vi "process_DAQ_NI.vi"(8 "error in (no error)":errorcluster) -> (0 "error out":errorcluster)   [LabVIEW 2010]
uses:
  typedefs/control_daq_enum.ctl
  typedefs/data_cluster.ctl
  typedefs/control_shutter_enum.ctl
  typedefs/main_state_enum.ctl
  typedefs/device_parameters.ctl
  typedefs/free_run_parameters.ctl
  typedefs/protocol_parameters.ctl
  <vilib>/DAQmx/read.llb/DAQmx Read (Analog 2D DBL NChan NSamp).vi
  <vilib>/daqmx/miscellaneous.llb/DAQmx Fill In Error Info.vi
panel:
  out "Onset":bool
  out "Waiting for trigger":bool
  out "Time [s]":dbl
  out "Repetition":dbl
  out "OFF":bool
  out "Post ON":bool
  out "ON":bool
  out "Pre ON":bool
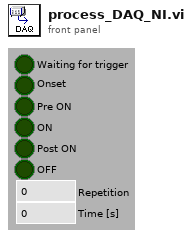
[diagram p1: front panel]
types:
  T1 = typedef "control_daq_enum.ctl" = enum16{"Init", "FreeRun", "Protocol", "Stop", "Quit"}
  T2 = cluster{"Control DAQ Enum":T1, "variant":variant}
  T3 = typedef "control_shutter_enum.ctl" = enum16{"Init", "Open", "Close", "Quit"}
  T4 = cluster{"Control shutter enum":T3, "variant":variant}
  T5 = typedef "data_cluster.ctl" = cluster{"t0":dbl, "dt":dbl, "Channels":dbl[][]}
  T6 = typedef "main_state_enum.ctl" = enum16{"Init", "Empty", "ParamsChanged", "Start", "Stop", "Abort", "Acquisition finished", "SetShutter", "Reset", "Error", "Quit"}
  T7 = typedef "device_parameters.ctl" = cluster{"Triggered?":bool, "Shutter channel":tag, "Acquisition channels":tag, "Acquisition sample rate":dbl, "Read chunk size":i32, "Stimulation channel":tag, "Stimulation sample rate":dbl}
  T8 = typedef "free_run_parameters.ctl" = cluster{"Stim onset":dbl, "Stim frequency":dbl, "Stim length":dbl, "Sync shutter to acquisition":bool}
  T9 = cluster{"Device parameters":T7, "Free run parameters":T8}
  T10 = typedef "protocol_parameters.ctl" = cluster{"Repetitions":dbl, "ON time":dbl, "OFF time":dbl, "Stim onset":dbl, "Stim frequency":dbl, "Pulse width":dbl, "Acquire before ON":dbl, "Acquire after ON":dbl, "Sync shutter to acquisition":bool}
  T11 = cluster{"Device parameters":T7, "Protocol parameters":T10}
  T12 = typedef "where_in_protocol_cluster.ctl" = cluster{"Onset":bool, "PreON":bool, "ON":bool, "PostON":bool, "OFF":bool, "Repetition":dbl, "Time":dbl}
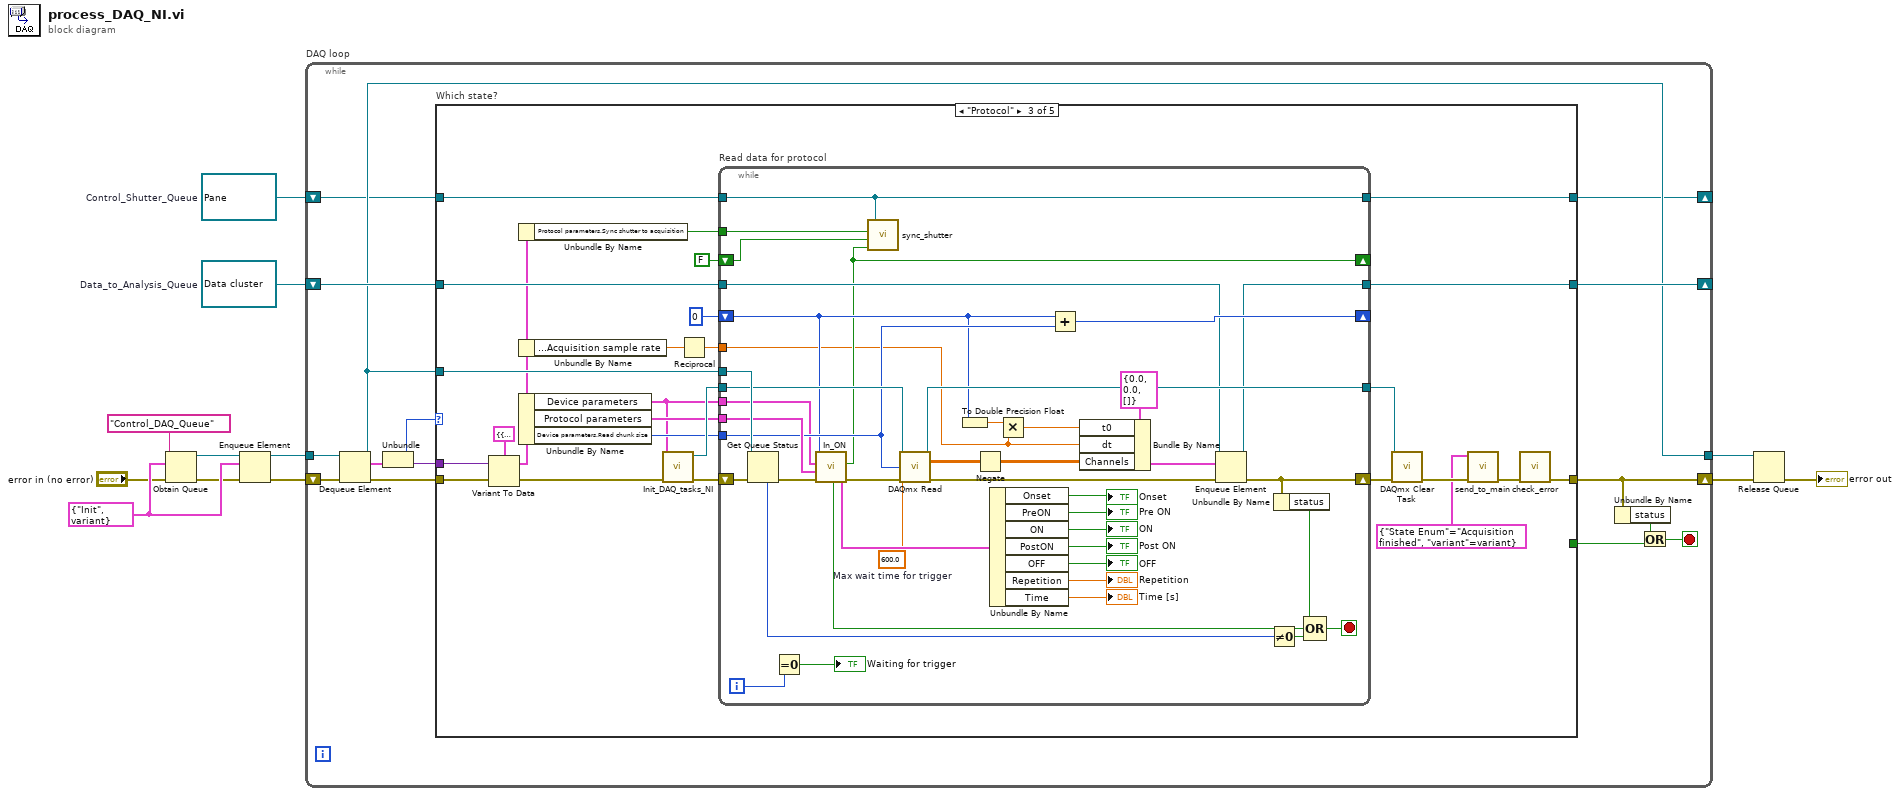
[diagram p0: block diagram]
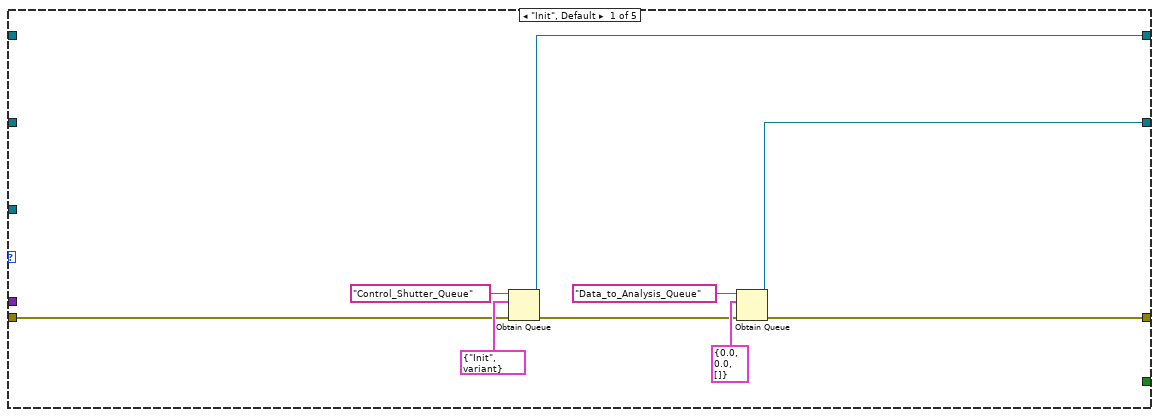
[diagram p2: hidden frame]
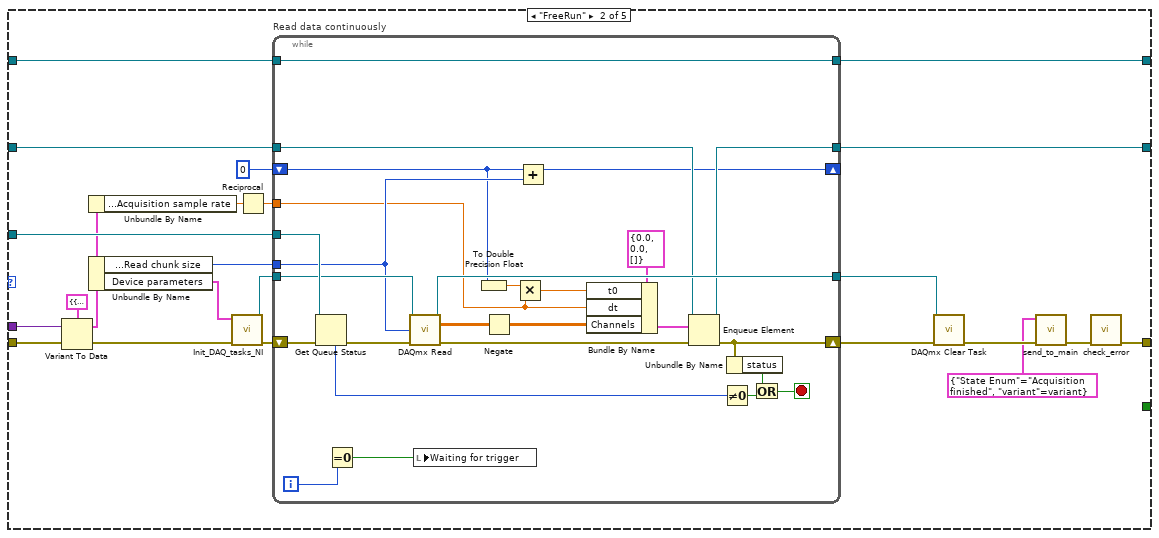
[diagram p3: hidden frame]
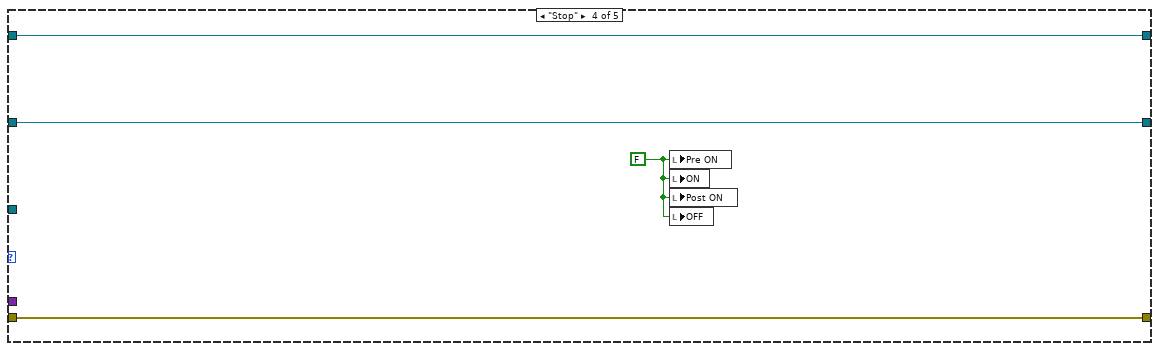
[diagram p4: hidden frame]
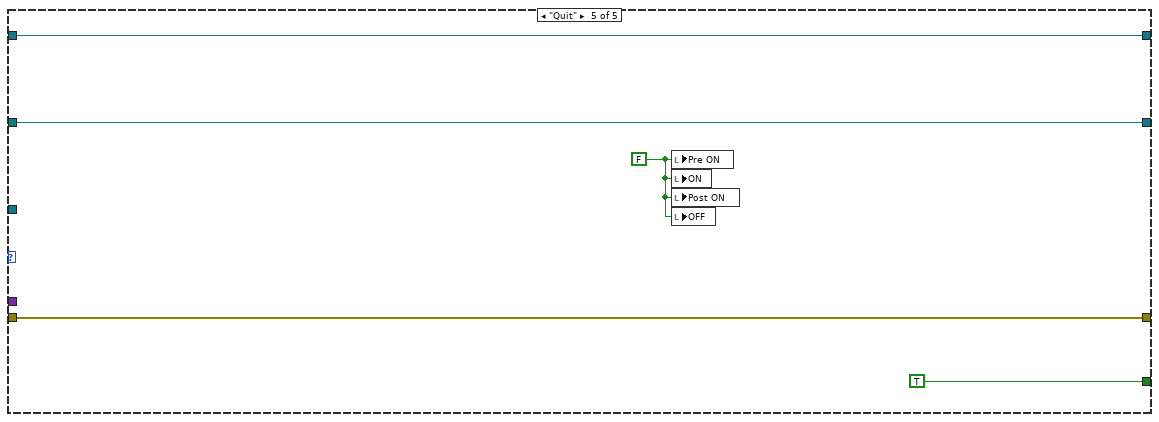
[diagram p5: hidden frame]
diagram:
  w1 = refnum<queue> refnum  # Control_Shutter_Queue
  w2 = refnum<queue> refnum  # Data_to_Analysis_Queue
  w12 = T2 {"Control DAQ Enum"=enum."Init", "variant"=variant} ("ControlDAQ state cluster")
  n1 = Obtain Queue(name (unnamed)="Control_DAQ_Queue", element data type=w12, error in (no error)="error in (no error)") -> (queue out=w8:refnum<queue>, error out=w10:errorcluster)  [unwired: 2 in, 1 out]
  n2 = Enqueue Element(queue=w8, element=w12, error in (no error)=w10) -> (queue out=w9:refnum<queue>, error out=w11:errorcluster)  [unwired: 1 in, 1 out]
  n3 = while "DAQ loop" {
    shift-right: [w21] -> w7
    shift-left: w11 -> [w26]
    tunnel: w9 -> [w27]
    tunnel: [w15] -> w6
    shift-right: [w16] -> _
    shift-left: w2 -> [w17]
    shift-right: [w13] -> _
    shift-left: w1 -> [w14]
    stop <- w19 stop-if-true
    n4 = Dequeue Element(queue=w27, error in (no error)=w26) -> (queue out=w15:refnum<queue>, element=w25:T2, error out=w23:errorcluster)  [unwired: 1 in, 1 out]
    n5 = Unbundle(w25) -> ("Control DAQ Enum"=w18:T1, "variant"=w24:variant)
    n6 = case "Which state?" shown="\"Protocol\"" w18 {
      tunnel: w15 -> [_ w59 w111 _ _]
      tunnel: w24 -> [_ w58 w110 _ _]
      tunnel: w23 -> [w28 w57 w109 w157 w161]
      tunnel: [w35 w45 w95 w157 w161] -> w21
      tunnel: [_ _ _ _ TRUE] -> w22
      tunnel: w17 -> [_ w48 w103 w156 w160]
      tunnel: [w34 w52 w102 w156 w160] -> w16
      tunnel: w14 -> [_ w43 w94 w155 w159]
      tunnel: [w29 w44 w90 w155 w159] -> w13
      frame "Init", Default {
        n7 = Obtain Queue(name (unnamed)="Control_Shutter_Queue", element data type=T4 {"Control shutter enum"=enum."Init", "variant"=variant}, error in (no error)=w28) -> (queue out=w29:refnum<queue>, error out=w32:errorcluster)  [unwired: 2 in, 1 out]
        n8 = Obtain Queue(name (unnamed)="Data_to_Analysis_Queue", element data type=T5 {"t0"=0.0, "dt"=0.0, "Channels"=[]} ("Data cluster"), error in (no error)=w32) -> (queue out=w34:refnum<queue>, error out=w35:errorcluster)  [unwired: 2 in, 1 out]
      }
      frame "FreeRun" {
        n9 = Variant To Data(error in=w57, Variant=w58, type=T9 {"Device parameters"={"Triggered?"=FALSE, "Shutter channel"="Dev1/port1/line3", "Acquisition channels"="Dev1/ai0:2", "Acquisition sample rate"=10000.0, "Read chunk size"=10, "Stimulation channel"="", "Stimulation sample rate"=100.0}, "Free run parameters"={"Stim onset"=5.0, "Stim frequency"=1.0, "Stim length"=0.001, "Sync shutter to acquisition"=TRUE}}) -> (error out=w40:errorcluster, data=w47:T9)
        n10 = Unbundle By Name(w47) -> ("Device parameters.Acquisition sample rate"=w42:dbl)
        n11 = Unbundle By Name(w47) -> ("Device parameters.Read chunk size"=w49:i32, "Device parameters"=w50:T7)
        n12 = call "Init_DAQ_tasks_NI.vi"("error in"=w40, "Device parameters"=w50) -> ("error out"=w56:errorcluster, "DAQ task out"=w55:refnum<k21>)  [unwired: 6 in]
        n13 = Reciprocal(x=w42) -> (1/x=w41:dbl)
        n14 = while "Read data continuously" {
          shift-right: [w80] -> w54
          shift-left: w56 -> [w81]
          tunnel: w59 -> [w85]
          tunnel: w55 -> [w78]
          tunnel: [w75] -> w53
          tunnel: [w74] -> w52
          tunnel: w49 -> [w69]
          tunnel: w48 -> [w73]
          tunnel: w41 -> [w66]
          shift-right: [w70] -> _
          shift-left: 0 -> [w68]
          tunnel: [w62] -> w44
          tunnel: w43 -> [w62]
          i -> [w61]
          stop <- w82 stop-if-true
          n15 = Get Queue Status(queue=w85, error in (no error)=w81) -> (error out=w76:errorcluster, # elements in queue=w84:i32)  [unwired: 1 in, 6 out]
          n16 = Equal To 0?(x=w61) -> (x = 0?=w60:bool)
          n17 = call-poly <vilib>:"DAQmx Read.vi"("task/channels in"=w78, "number of samples per channel"=w69, "error in"=w76) -> ("task out"=w75:refnum<k21>, "data"=w64:dbl[][], "error out"=w77:errorcluster)  [unwired: 10 in]
          n18 = local write "Waiting for trigger"(w60) -> ()
          n19 = To Double Precision Float(number=w68) -> (double precision float=w67:dbl)
          n20 = Negate(x=w64) -> (-x=w63:dbl[][])
          n21 = Multiply(x=w67, y=w66) -> (x*y=w65:dbl)
          n22 = Add(x=w68, y=w69) -> (x+y=w70:i32)
          n23 = Bundle By Name(cluster=T5 {"t0"=0.0, "dt"=0.0, "Channels"=[]} ("Data cluster"), "t0"=w65, "dt"=w66, "Channels"=w63) -> (w71:T5)
          n24 = Enqueue Element(queue=w73, element=w71, error in (no error)=w77) -> (queue out=w74:refnum<queue>, error out=w80:errorcluster)  [unwired: 1 in, 1 out]
          n25 = Not Equal To 0?(x=w84) -> (x != 0?=w83:bool)
          n26 = Unbundle By Name(w80) -> ("status"=w79:bool)
          n27 = Or(x=w79, y=w83) -> (x .or. y?=w82:bool)
        }
        n28 = call <vilib>:"DAQmx Clear Task.vi"("task in"=w53, "error in"=w54) -> ("error out"=w39:errorcluster)  [unwired: 13 in]
        n29 = call "send_to_main.vi"("error in (no error)"=w39, "Main state cluster"=cluster{"State Enum":T6, "variant":variant} {"State Enum"=enum."Acquisition finished", "variant"=variant} ("element")) -> ("error out"=w38:errorcluster)  [unwired: 9 in]
        n30 = call "check_error.vi"("error in"=w38) -> ("error out"=w45:errorcluster)  [unwired: 10 in]
      }
      frame "Protocol" {
        n31 = Variant To Data(error in=w109, Variant=w110, type=T11 {"Device parameters"={"Triggered?"=FALSE, "Shutter channel"="", "Acquisition channels"="", "Acquisition sample rate"=100.0, "Read chunk size"=0, "Stimulation channel"="", "Stimulation sample rate"=0.0}, "Protocol parameters"={"Repetitions"=1.0, "ON time"=40.0, "OFF time"=120.0, "Stim onset"=5.0, "Stim frequency"=1.0, "Pulse width"=1.0, "Acquire before ON"=1.0, "Acquire after ON"=0.0, "Sync shutter to acquisition"=FALSE}}) -> (error out=w91:errorcluster, data=w93:T11)
        n32 = Unbundle By Name(w93) -> ("Protocol parameters.Sync shutter to acquisition"=w92:bool)
        n33 = Unbundle By Name(w93) -> ("Device parameters.Acquisition sample rate"=w97:dbl)
        n34 = Unbundle By Name(w93) -> ("Device parameters"=w99:T7, "Protocol parameters"=w101:T10, "Device parameters.Read chunk size"=w100:i32)
        n35 = call "Init_DAQ_tasks_NI.vi"("error in"=w91, "Device parameters"=w99) -> ("error out"=w108:errorcluster, "DAQ task out"=w107:refnum<k21>)  [unwired: 6 in]
        n36 = Reciprocal(x=w97) -> (1/x=w96:dbl)
        n37 = while "Read data for protocol" {
          shift-right: [w143] -> w106
          shift-left: w108 -> [w151]
          tunnel: w111 -> [w153]
          tunnel: w107 -> [w150]
          tunnel: [w149] -> w105
          shift-right: [w148] -> _
          shift-left: 0 -> [w138]
          tunnel: w103 -> [w147]
          tunnel: [w146] -> w102
          tunnel: w99 -> [w136]
          tunnel: w101 -> [w142]
          tunnel: w100 -> [w141]
          tunnel: w96 -> [w126]
          tunnel: w94 -> [w119]
          shift-right: [w129] -> _
          shift-left: FALSE ("Do acquire") -> [w131]
          tunnel: w92 -> [w130]
          tunnel: [w119] -> w90
          i -> [w114]
          stop <- w134 stop-if-true
          w115 = 600.0  # Max wait time for trigger
          n38 = Get Queue Status(queue=w153, error in (no error)=w151) -> (error out=w145:errorcluster, # elements in queue=w152:i32)  [unwired: 1 in, 6 out]
          n39 = Equal To 0?(x=w114) -> (x = 0?=→"Waiting for trigger":bool)
          n40 = call "In_ON.vi"("error in"=w145, "Protocol parameters"=w142, "Device parameters"=w136, "Read position"=w138) -> ("error out"=w144:errorcluster, "Finished?"=w132:bool, "Do acquire"=w129:bool, "Where"=w125:T12)  [unwired: 4 in]
          n41 = call "sync_shutter.vi"("Do acquire?"=w129, "Old acquire state"=w131, "Sync shutter to acquisition"=w130, "Control_Shutter_Queue"=w119) -> ()  [unwired: 1 in]
          n42 = call-poly <vilib>:"DAQmx Read.vi"("task/channels in"=w150, "number of samples per channel"=w141, "timeout"=w115, "error in"=w144) -> ("task out"=w149:refnum<k21>, "data"=w122:dbl[][], "error out"=w140:errorcluster)  [unwired: 9 in]
          n43 = To Double Precision Float(number=w138) -> (double precision float=w128:dbl)
          n44 = Negate(x=w122) -> (-x=w121:dbl[][])
          n45 = Unbundle By Name(w125) -> ("Onset"=→"Onset":bool, "PreON"=→"Pre ON":bool, "ON"=→"ON":bool, "PostON"=→"Post ON":bool, "OFF"=→"OFF":bool, "Repetition"=→"Repetition":dbl, "Time"=→"Time [s]":dbl)
          n46 = Multiply(x=w128, y=w126) -> (x*y=w127:dbl)
          n47 = Add(x=w138, y=w141) -> (x+y=w148:i32)
          n48 = Bundle By Name(cluster=T5 {"t0"=0.0, "dt"=0.0, "Channels"=[]} ("Data cluster"), "t0"=w127, "dt"=w126, "Channels"=w121) -> (w137:T5)
          n49 = Enqueue Element(queue=w147, element=w137, error in (no error)=w140) -> (queue out=w146:refnum<queue>, error out=w143:errorcluster)  [unwired: 1 in, 1 out]
          n50 = Not Equal To 0?(x=w152) -> (x != 0?=w133:bool)
          n51 = Unbundle By Name(w143) -> ("status"=w135:bool)
          n52 = Compound Arithmetic op=OR(w135, w132, w133) -> (w134:bool)
        }
        n53 = call <vilib>:"DAQmx Clear Task.vi"("task in"=w105, "error in"=w106) -> ("error out"=w88:errorcluster)  [unwired: 13 in]
        n54 = call "send_to_main.vi"("error in (no error)"=w88, "Main state cluster"=cluster{"State Enum":T6, "variant":variant} {"State Enum"=enum."Acquisition finished", "variant"=variant} ("element")) -> ("error out"=w87:errorcluster)  [unwired: 9 in]
        n55 = call "check_error.vi"("error in"=w87) -> ("error out"=w95:errorcluster)  [unwired: 10 in]
      }
      frame "Stop" {
        w154 = FALSE ("Pre ON")
        n56 = local write "Pre ON"(w154) -> ()
        n57 = local write "ON"(w154) -> ()
        n58 = local write "Post ON"(w154) -> ()
        n59 = local write "OFF"(w154) -> ()
      }
      frame "Quit" {
        w158 = FALSE ("Pre ON")
        n60 = local write "Pre ON"(w158) -> ()
        n61 = local write "ON"(w158) -> ()
        n62 = local write "Post ON"(w158) -> ()
        n63 = local write "OFF"(w158) -> ()
      }
    }
    n64 = Unbundle By Name(w21) -> ("status"=w20:bool)
    n65 = Or(x=w20, y=w22) -> (x .or. y?=w19:bool)
  }
  n66 = Release Queue(queue=w6, error in (no error)=w7) -> (error out=→"error out":errorcluster)  [unwired: 1 in, 2 out]
